vi "Constants.vi"() -> ()   [LabVIEW 2015, in "Waveform-Processing-Custom-Device Shared.lvlib"]
doc: "Use this Global VI to access the GUIDs assigned to the page resources of the Custom Device."
uses:
  Waveform-Processing-Custom-Device Shared.lvlib
panel:
  in  "Tab Control":enum32{"GUIDS", "Constants", "Properties"}(tab)
  in  "Running Average Parameter Channel GUID":string="843E991B-7832-4F2E-8B2E-6013407FE1A1"
  in  "Scaled Waveform Parameter Channel GUID":string="BEEA8E39-933C-4D5D-BDD4-EE2FB842ECD5"
  in  "Scaled Waveform Results Channel GUID":string="6554AA7C-9F21-4A98-9F8F-BEAFBF9477D8"
  in  "Single Point Results Channel GUID":string="D679E461-A382-4B26-A9C7-0EC8D0A53C2E"
  in  "Running Average Results Channel GUID":string="0FFE099E-DEB7-4308-AE45-614A1A79D1E8"
  in  "Waveform-Processing-Custom-Device Disabled":string="7b547a45-b3bf-4a70-a525-6bc55fa12b7c"
  in  "Waveform Results Section GUID":string="e38e89f1-3d1b-4012-b75e-d54b3a46b12e"
  in  "Running Average Settings GUID":string="98bae003-a8c4-4cad-9e5d-6f3690f27bc7"
  in  "Waveform-Processing-Custom-Device":string="2e5751d4-f26f-4961-8df7-f46ae00d1276"
  in  "Scaled Waveform Parameters Channel Group":string="Scaled Waveform Parameters Channel Group"
  in  "Running Average Parameters Channel Group":string="Running Average Parameters Channel Group"
  in  "Single Point Result Channel Group":string="Single Point Result Channel Group"
  in  "Running Average Result Channel Group":string="Running Average Result Channel Group"
  in  "Waveform Processing Custom Device Name":string="Waveform Processing Custom Device"
  in  "Running Average Period":string="Running Average Period"
  in  "Running Average Settings":string="Running Average Settings"
  in  "Scaled.Waveform.Settings.Scale":string="ScaledWaveformScale"
  in  "Scaled.Waveform.Enabled":string="ScaledWaveformEnabled"
  in  "Result.Section.Scaled.Waveform.Channel":string="ResultScaledWaveform"
  in  "CD.TaskRate":string="TaskRate"
  in  "CD.BufferSamples":string="BufferSamples"
  in  "CD.TaskDependencyRef":string="TaskDependencyRef"
  in  "CD.BufferSeconds":string="BufferSeconds"
  in  "CD.SelectedWaveforms":string="SelectedWfms"
  in  "CD.AvailableWfms":string="AvailableWfms"
  in  "Result.Section.Single.Point.Channel":string="ResultSinglePoint"
  in  "Running.Average.Settings.Period.Channel":string="RunningAveragePeriod"
  in  "Result.Section.Running.Average.Channel":string="ResultRunningAverage"
  in  "Single.Point.Enabled":string="SinglePointEnabled"
  in  "Running.Average.Enabled":string="RunningAverageEnabled"
  in  "Compiled.Settings":string="CompiledSettings"
  in  "Result.Section.Wfm.Dependency":string="WfmDependency"
  in  "CD.TaskDependency":string="TaskDependency"
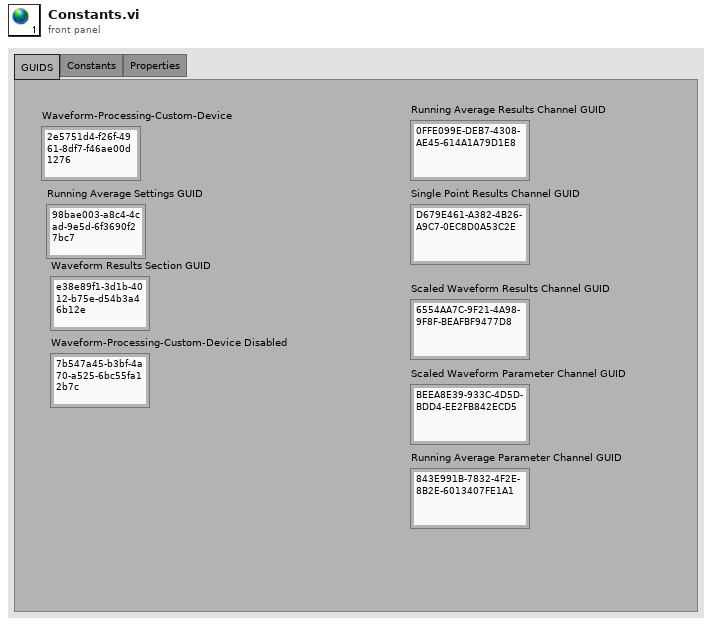
[diagram p1: front panel]
diagram:
